vi "Control Panel.vi"(8 "error in (no error)":errorcluster, 11 "Fake MicrowaveAmp in":refnum<class "MicrowaveAmp.lvclass">) -> (0 "error out":errorcluster, 3 "Fake MicrowaveAmp out":refnum<class "MicrowaveAmp.lvclass">)   [LabVIEW 2009, in "MicrowaveAmp.lvclass"]
doc: "(Dynamic) A user-level application that simulates the physical front panel of the Instrument. Provide the user with buttons to manually control features of the instrument, and provide indicators of its current state."
uses:
  MicrowaveAmp.lvclass
  Utility Classes/Scannable/Scannable.lvclass
  MicrowaveAmp.lvclass/MicrowaveAmp.ctl
panel:
  in  "Copy actual to set":bool
  in  "Populate fields with member data":bool
  in  "Read Remaining Time Delay":bool
  in  "Read Amplifier Status/Mode":bool
  in  "Standby":bool
  in  "stop":bool
  out "Mode":u16(ring) items=["SLEEP", "WARM-UP", "STANDBY", "OPERATE", "FAULT"]
  in  "Operate":bool
  in  "Read Reverse Power Out (W)":bool
  in  "Read Reverse Power Out (dBm)":bool
  in  "Read Forward Power Out (W)":bool
  in  "Read Forward Power out (dBm)":bool
  in  "Read Gain":bool
  in  "Set Gain":bool
  out "Remaining Heater Delay Time":dbl[unit]
  out "Reverse Power Out (dBm)":dbl
  out "Reverse Power Out (W)":dbl[unit]
  out "Forward Power Out (dBm)":dbl
  out "Forward Power Out (W)":dbl[unit]
  out "Gain (%)":dbl
  in  "GainSet":dbl
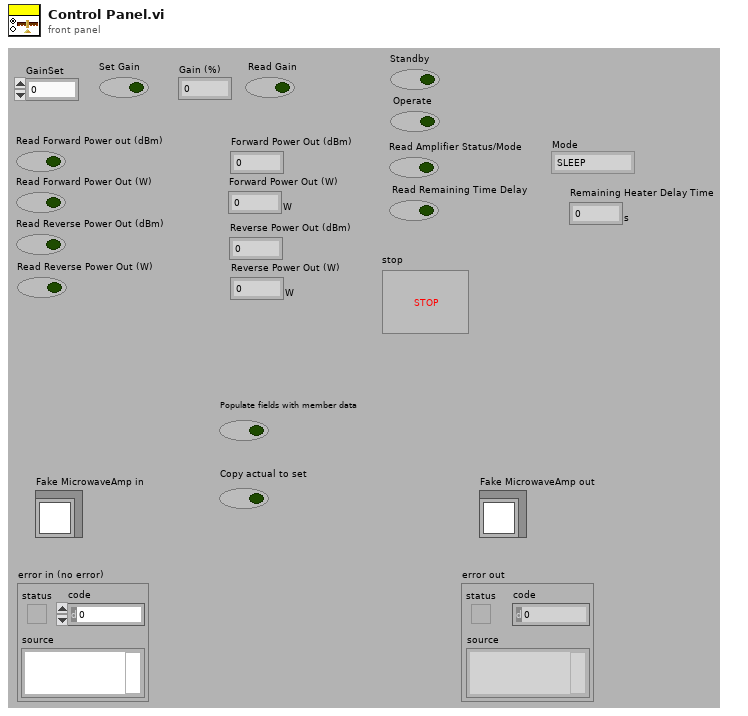
[diagram p1: front panel]
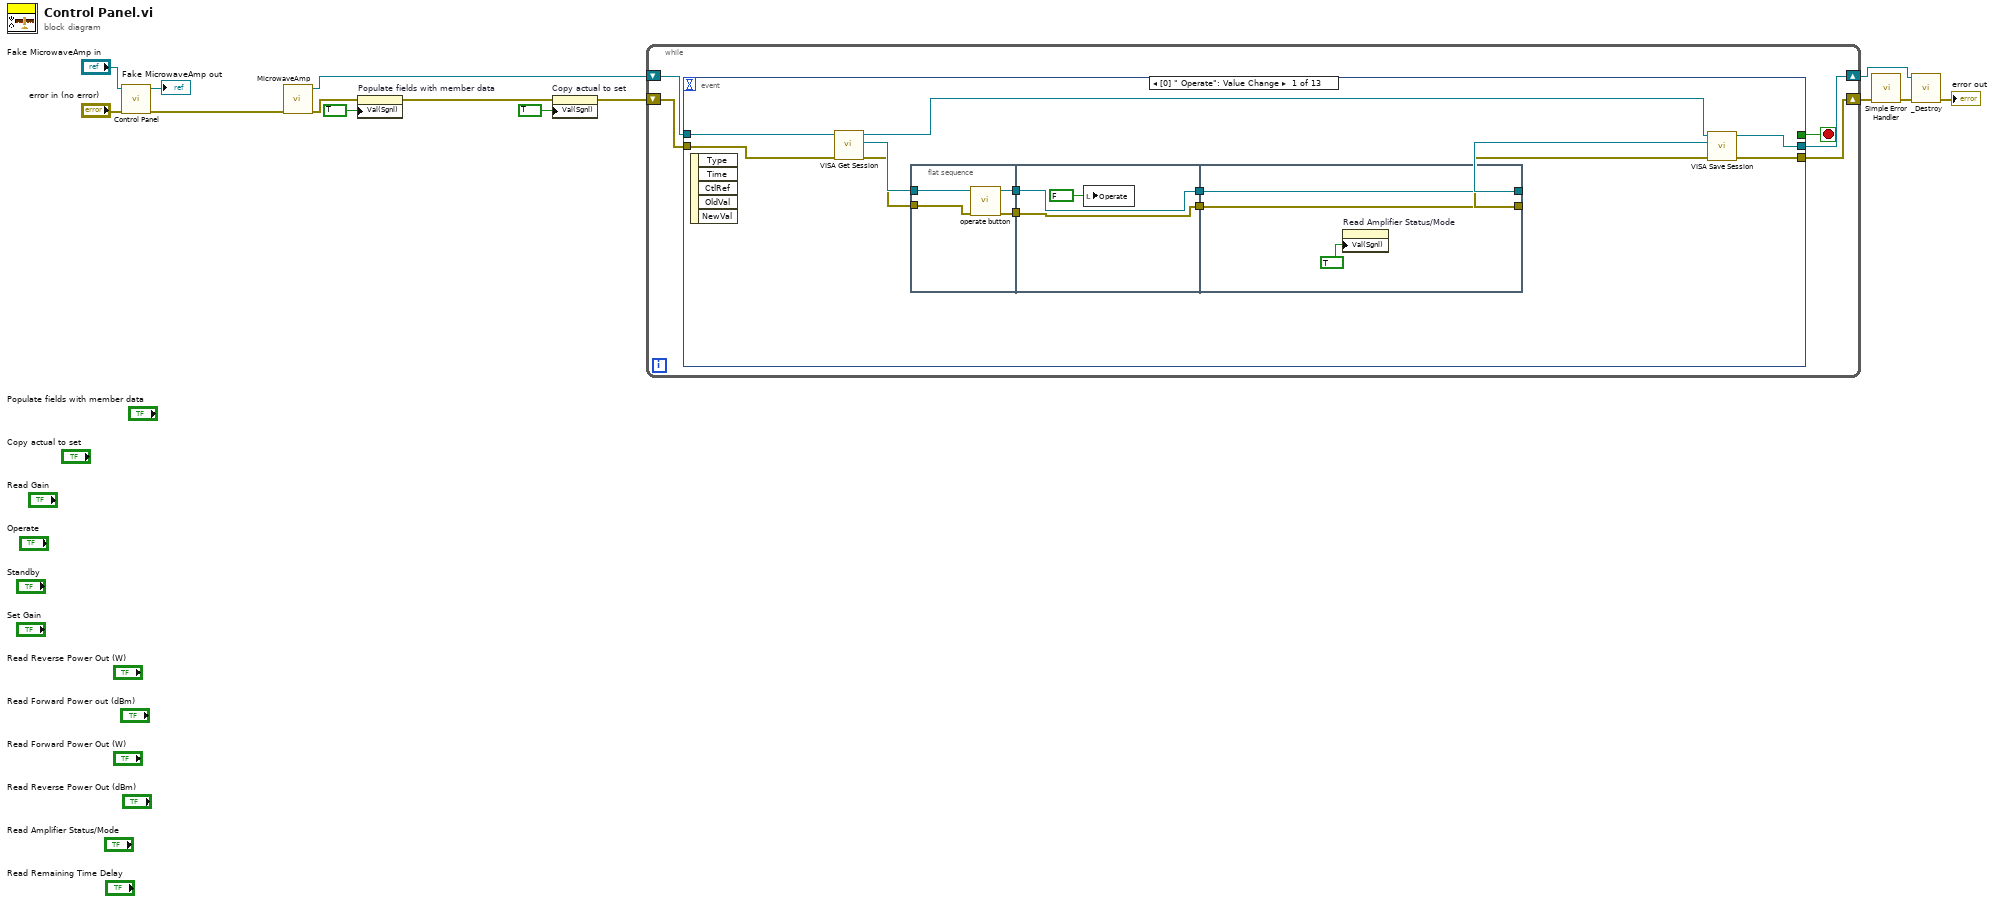
[diagram p0: block diagram]
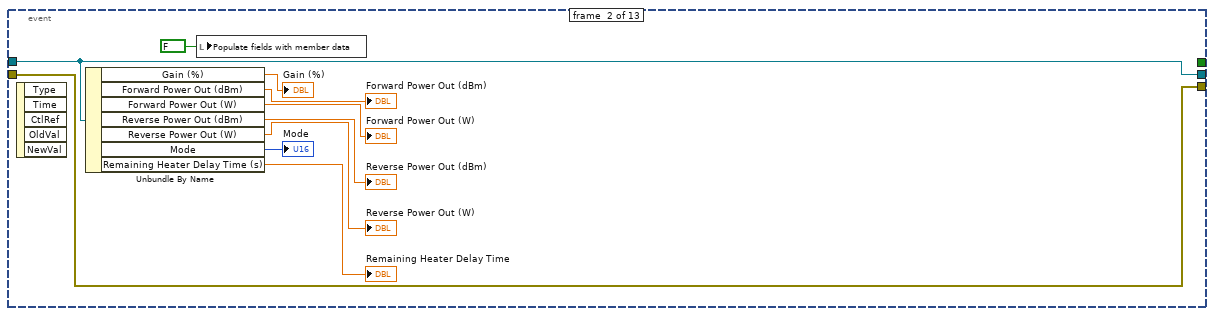
[diagram p2: hidden frame]
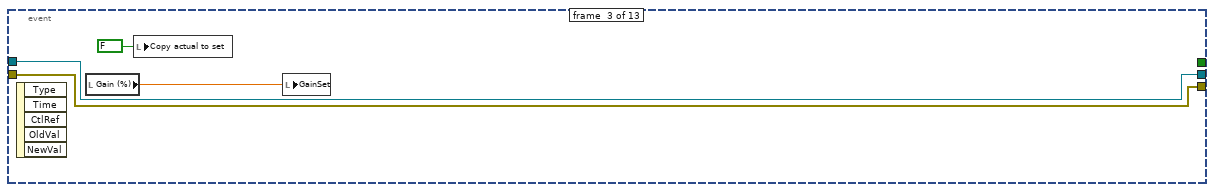
[diagram p3: hidden frame]
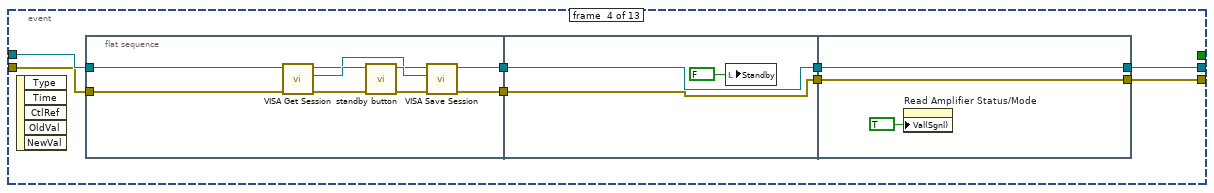
[diagram p4: hidden frame]
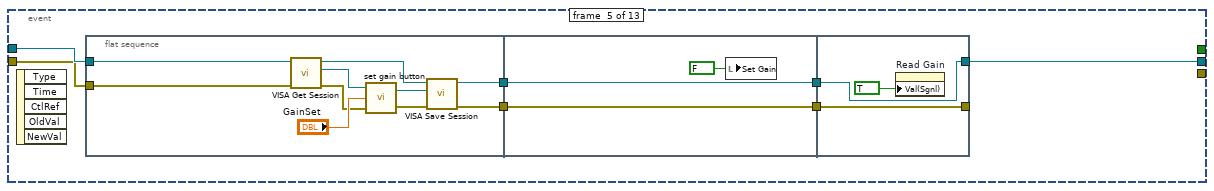
[diagram p5: hidden frame]
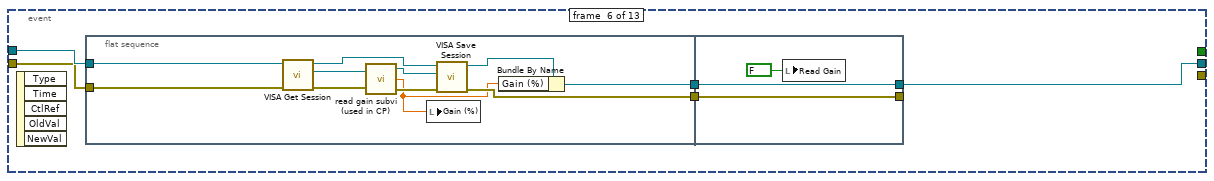
[diagram p6: hidden frame]
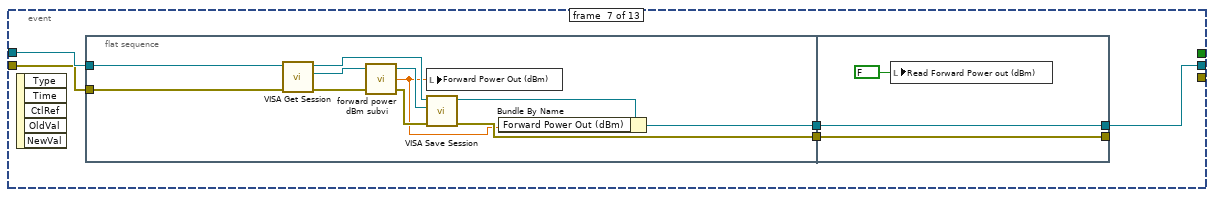
[diagram p7: hidden frame]
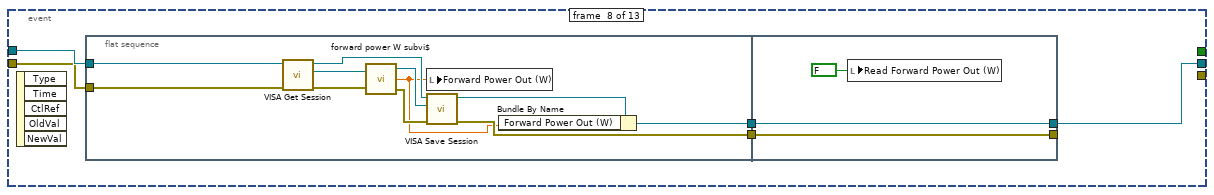
[diagram p8: hidden frame]
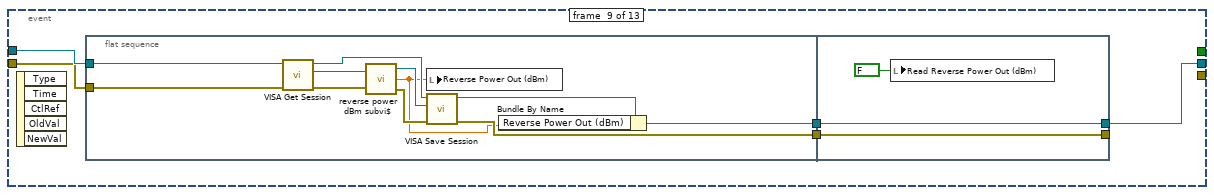
[diagram p9: hidden frame]
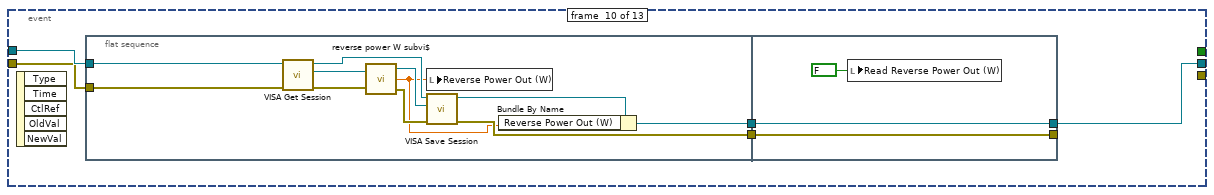
[diagram p10: hidden frame]
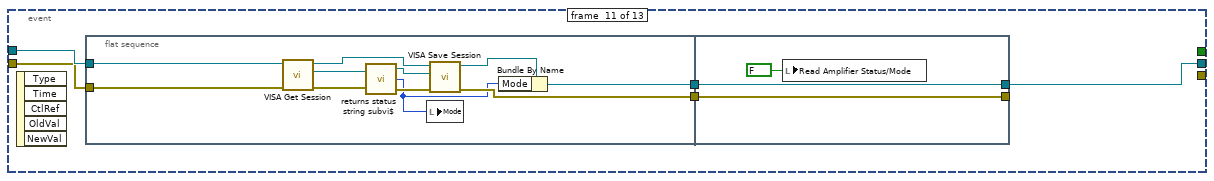
[diagram p11: hidden frame]
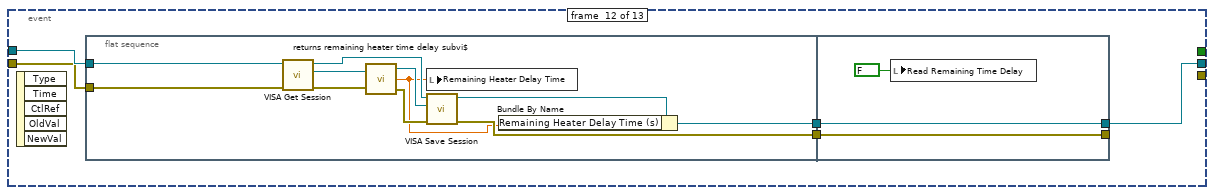
[diagram p12: hidden frame]
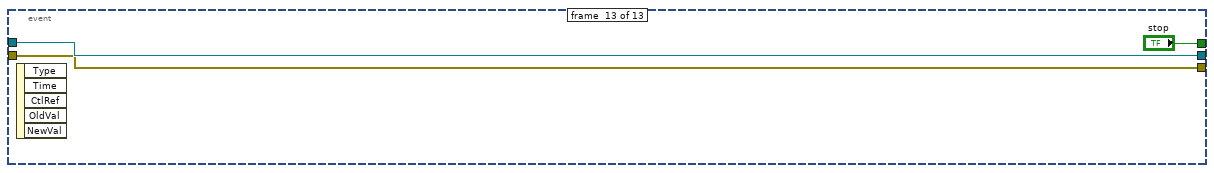
[diagram p13: hidden frame]
diagram:
  n1 = call-parent "Control Panel.vi"("error in (no error)"="error in (no error)", "Instrument in"="Fake MicrowaveAmp in") -> ("error out"=w9:errorcluster, "Instrument out"=→"Fake MicrowaveAmp out":refnum<class "MicrowaveAmp.lvclass">)  [unwired: 8 in]
  n2 = call "MicrowaveAmp.vi"("error in (no error)"=w9) -> ("error out"=w10:errorcluster, "MicrowaveAmp out"=w1:refnum<class "MicrowaveAmp.lvclass">)  [unwired: 9 in]
  n3 = property on="Populate fields with member data" class="Bool (strict)"(error in=w10, "Val(Sgnl)"=TRUE ("Value (Signaling)")) -> (error out=w11:errorcluster)  [unwired: 1 in, 1 out]
  n4 = property on="Copy actual to set" class="Bool (strict)"(error in=w11, "Val(Sgnl)"=TRUE ("Value (Signaling)")) -> (error out=w2:errorcluster)  [unwired: 1 in, 1 out]
  n5 = while {
    shift-right: [w19] -> w5
    shift-left: w2 -> [w16]
    shift-right: [w17] -> w8
    shift-left: w1 -> [w15]
    stop <- w18 stop-if-true
    n6 = event shown="[0] \" Operate\": Value Change" {
      selector: _ -> [_ _ _ _ _ _ _ _ _ _ _ _ _]
      dyn-events: _ -> [_ _ _ _ _ _ _ _ _ _ _ _ _]
      timeout: _ -> [_ _ _ _ _ _ _ _ _ _ _ _ _]
      tunnel: w16 -> [w23 w52 w55 w59 w83 w105 w122 w141 w160 w179 w198 w219 w236]
      tunnel: [w25 w52 w55 w63 _ _ _ _ _ _ _ _ w236] -> w19
      tunnel: [_ _ _ _ _ _ _ _ _ _ _ _ "stop"] -> w18
      tunnel: w15 -> [w29 w51 w56 w60 w84 w106 w125 w144 w163 w182 w201 w220 w237]
      tunnel: [w26 w51 w56 w61 w82 w104 w124 w143 w162 w181 w200 w218 w237] -> w17
      event #0 {
        n7 = event-data() -> ()  [unwired: 1 in, 5 out]
        n8 = call-dynamic "VISA Get Session.vi"("error in (no error)"=w23, "Instrument.lvclass in"=w29) -> ("error out"=w22:errorcluster, "VISA Resource Name"=w30:refnum<visa-resource-name>, "Instrument.lvclass out"=w27:refnum<class "MicrowaveAmp.lvclass">)  [unwired: 7 out]
        n9 = flat-sequence {
          tunnel: [w36] -> w32
          tunnel: [w35] -> w31
          tunnel: w22 -> [w34]
          tunnel: w30 -> [w33]
          tunnel: w32 -> [w38]
          tunnel: w31 -> [w37]
          tunnel: [w38] -> w21
          tunnel: [w37] -> w20
          tunnel: [w41] -> w24
          tunnel: [w42] -> w28
          tunnel: w21 -> [w42]
          tunnel: w20 -> [w41]
          frame #0 {
            n10 = call "operate button.vi"("error in (no error)"=w34, "VISA resource name"=w33) -> ("error out"=w35:errorcluster, "VISA resource name out"=w36:refnum<visa-resource-name>)  [unwired: 8 in]
          }
          frame #1 {
            n11 = local write "Operate"(FALSE ("Operate")) -> ()
          }
          frame #2 {
            n12 = property on="Read Amplifier Status/Mode" class="Bool (strict)"("Val(Sgnl)"=TRUE ("Value (Signaling)")) -> ()  [unwired: 2 in, 2 out]
          }
        }
        n13 = call-dynamic "VISA Save Session.vi"("error in (no error)"=w24, "VISA Resource Name"=w28, "Instrument.lvclass in"=w27) -> ("error out"=w25:errorcluster, "Instrument.lvclass out"=w26:refnum<class "MicrowaveAmp.lvclass">)  [unwired: 7 out]
      }
      event #1 {
        n14 = event-data() -> ()  [unwired: 1 in, 5 out]
        n15 = Unbundle By Name(w51) -> ("Gain (%)"=→"Gain (%)":dbl, "Forward Power Out (dBm)"=→"Forward Power Out (dBm)":dbl, "Forward Power Out (W)"=→"Forward Power Out (W)":dbl[unit], "Reverse Power Out (dBm)"=→"Reverse Power Out (dBm)":dbl, "Reverse Power Out (W)"=→"Reverse Power Out (W)":dbl[unit], "Mode"=→"Mode":u16, "Remaining Heater Delay Time (s)"=→"Remaining Heater Delay Time":dbl[unit])
        n16 = local write "Populate fields with member data"(FALSE ("Populate fields with member data")) -> ()
      }
      event #2 {
        n17 = event-data() -> ()  [unwired: 1 in, 5 out]
        n18 = local read "Gain (%)"() -> (w53:dbl)
        n19 = local write "Copy actual to set"(FALSE ("Copy actual to set")) -> ()
        n20 = local write "GainSet"(w53) -> ()
      }
      event #3 {
        n21 = event-data() -> ()  [unwired: 1 in, 5 out]
        n22 = flat-sequence {
          tunnel: [w72] -> w64
          tunnel: [w71] -> w62
          tunnel: w60 -> [w69]
          tunnel: w59 -> [w68]
          tunnel: w64 -> [w75]
          tunnel: w62 -> [w74]
          tunnel: [w75] -> w58
          tunnel: [w74] -> w57
          tunnel: [w78] -> w61
          tunnel: [w79] -> w63
          tunnel: w58 -> [w79]
          tunnel: w57 -> [w78]
          frame #0 {
            n23 = call-dynamic "VISA Get Session.vi"("error in (no error)"=w68, "Instrument.lvclass in"=w69) -> ("error out"=w67:errorcluster, "VISA Resource Name"=w66:refnum<visa-resource-name>, "Instrument.lvclass out"=w65:refnum<class "MicrowaveAmp.lvclass">)  [unwired: 7 out]
            n24 = call "standby button.vi"("error in (no error)"=w67, "VISA resource name"=w66) -> ("error out"=w70:errorcluster, "VISA resource name out"=w73:refnum<visa-resource-name>)  [unwired: 8 in]
            n25 = call-dynamic "VISA Save Session.vi"("error in (no error)"=w70, "VISA Resource Name"=w73, "Instrument.lvclass in"=w65) -> ("error out"=w72:errorcluster, "Instrument.lvclass out"=w71:refnum<class "MicrowaveAmp.lvclass">)  [unwired: 7 out]
          }
          frame #1 {
            n26 = local write "Standby"(FALSE ("Operate")) -> ()
          }
          frame #2 {
            n27 = property on="Read Amplifier Status/Mode" class="Bool (strict)"("Val(Sgnl)"=TRUE ("Value (Signaling)")) -> ()  [unwired: 2 in, 2 out]
          }
        }
      }
      event #4 {
        n28 = event-data() -> ()  [unwired: 1 in, 5 out]
        n29 = flat-sequence {
          tunnel: [w89] -> w86
          tunnel: w84 -> [w95]
          tunnel: w83 -> [w94]
          tunnel: [w92] -> w80
          tunnel: w86 -> [w98]
          tunnel: [w98] -> w85
          tunnel: [w97] -> w81
          tunnel: w80 -> [w97]
          tunnel: [w102] -> _
          tunnel: w85 -> [w102]
          tunnel: [w100] -> w82
          tunnel: w81 -> [w100]
          frame #0 {
            n30 = call-dynamic "VISA Get Session.vi"("error in (no error)"=w94, "Instrument.lvclass in"=w95) -> ("error out"=w91:errorcluster, "VISA Resource Name"=w87:refnum<visa-resource-name>, "Instrument.lvclass out"=w93:refnum<class "MicrowaveAmp.lvclass">)  [unwired: 7 out]
            n31 = call "set gain button.vi"("error in (no error)"=w91, "Gain"="GainSet", "VISA resource name"=w87) -> ("error out"=w90:errorcluster, "VISA resource name out"=w88:refnum<visa-resource-name>)
            n32 = call-dynamic "VISA Save Session.vi"("error in (no error)"=w90, "VISA Resource Name"=w88, "Instrument.lvclass in"=w93) -> ("error out"=w89:errorcluster, "Instrument.lvclass out"=w92:refnum<class "MicrowaveAmp.lvclass">)  [unwired: 7 out]
          }
          frame #1 {
            n33 = local write "Set Gain"(FALSE ("Set Gain")) -> ()
          }
          frame #2 {
            n34 = property on="Read Gain" class="Bool (strict)"("Val(Sgnl)"=TRUE ("Value (Signaling)")) -> ()  [unwired: 2 in, 2 out]
          }
        }
      }
      event #5 {
        n35 = event-data() -> ()  [unwired: 1 in, 5 out]
        n36 = flat-sequence {
          tunnel: [w114] -> w107
          tunnel: w106 -> [w118]
          tunnel: w105 -> [w117]
          tunnel: [w108] -> w103
          tunnel: [w120] -> _
          tunnel: w107 -> [w120]
          tunnel: [w119] -> w104
          tunnel: w103 -> [w119]
          frame #0 {
            n37 = call-dynamic "VISA Get Session.vi"("error in (no error)"=w117, "Instrument.lvclass in"=w118) -> ("error out"=w116:errorcluster, "VISA Resource Name"=w113:refnum<visa-resource-name>, "Instrument.lvclass out"=w111:refnum<class "MicrowaveAmp.lvclass">)  [unwired: 7 out]
            n38 = call "read gain subvi (used in CP).vi"("VISA resource name"=w113, "error in (no error)"=w116) -> ("VISA resource name out"=w112:refnum<visa-resource-name>, "Gain (%)"=w110:dbl, "error out"=w115:errorcluster)
            n39 = local write "Gain (%)"(w110) -> ()
            n40 = call-dynamic "VISA Save Session.vi"("error in (no error)"=w115, "VISA Resource Name"=w112, "Instrument.lvclass in"=w111) -> ("error out"=w114:errorcluster, "Instrument.lvclass out"=w109:refnum<class "MicrowaveAmp.lvclass">)  [unwired: 7 out]
            n41 = Bundle By Name(cluster=w109, "Gain (%)"=w110) -> (w108:refnum<class "MicrowaveAmp.lvclass">)
          }
          frame #1 {
            n42 = local write "Read Gain"(FALSE ("Read Gain")) -> ()
          }
        }
      }
      event #6 {
        n43 = event-data() -> ()  [unwired: 1 in, 5 out]
        n44 = flat-sequence {
          tunnel: [w132] -> w126
          tunnel: w125 -> [w137]
          tunnel: [w127] -> w123
          tunnel: w122 -> [w135]
          tunnel: [w140] -> _
          tunnel: w126 -> [w140]
          tunnel: [w138] -> w124
          tunnel: w123 -> [w138]
          frame #0 {
            n45 = call-dynamic "VISA Get Session.vi"("error in (no error)"=w135, "Instrument.lvclass in"=w137) -> ("error out"=w134:errorcluster, "VISA Resource Name"=w131:refnum<visa-resource-name>, "Instrument.lvclass out"=w136:refnum<class "MicrowaveAmp.lvclass">)  [unwired: 7 out]
            n46 = call "forward power dBm subvi.vi"("error in (no error)"=w134, "VISA resource name"=w131) -> ("error out"=w133:errorcluster, "forward power (dBm)"=w129:dbl, "VISA resource name out"=w130:refnum<visa-resource-name>)  [unwired: 1 in]
            n47 = local write "Forward Power Out (dBm)"(w129) -> ()
            n48 = call-dynamic "VISA Save Session.vi"("error in (no error)"=w133, "VISA Resource Name"=w130, "Instrument.lvclass in"=w136) -> ("error out"=w132:errorcluster, "Instrument.lvclass out"=w128:refnum<class "MicrowaveAmp.lvclass">)  [unwired: 7 out]
            n49 = Bundle By Name(cluster=w128, "Forward Power Out (dBm)"=w129) -> (w127:refnum<class "MicrowaveAmp.lvclass">)
          }
          frame #1 {
            n50 = local write "Read Forward Power out (dBm)"(FALSE ("Read Forward Power out (dBm)")) -> ()
          }
        }
      }
      event #7 {
        n51 = event-data() -> ()  [unwired: 1 in, 5 out]
        n52 = flat-sequence {
          tunnel: [w150] -> w145
          tunnel: w144 -> [w155]
          tunnel: [w146] -> w142
          tunnel: w141 -> [w153]
          tunnel: [w159] -> _
          tunnel: w145 -> [w159]
          tunnel: [w157] -> w143
          tunnel: w142 -> [w157]
          frame #0 {
            n53 = call-dynamic "VISA Get Session.vi"("error in (no error)"=w153, "Instrument.lvclass in"=w155) -> ("error out"=w152:errorcluster, "VISA Resource Name"=w156:refnum<visa-resource-name>, "Instrument.lvclass out"=w154:refnum<class "MicrowaveAmp.lvclass">)  [unwired: 7 out]
            n54 = call "forward power W subvi$.vi"("VISA resource name"=w156, "error in (no error)"=w152) -> ("VISA resource name out"=w149:refnum<visa-resource-name>, "foward power (W)"=w148:dbl[unit], "error out"=w151:errorcluster)
            n55 = local write "Forward Power Out (W)"(w148) -> ()
            n56 = call-dynamic "VISA Save Session.vi"("error in (no error)"=w151, "VISA Resource Name"=w149, "Instrument.lvclass in"=w154) -> ("error out"=w150:errorcluster, "Instrument.lvclass out"=w147:refnum<class "MicrowaveAmp.lvclass">)  [unwired: 7 out]
            n57 = Bundle By Name(cluster=w147, "Forward Power Out (W)"=w148) -> (w146:refnum<class "MicrowaveAmp.lvclass">)
          }
          frame #1 {
            n58 = local write "Read Forward Power Out (W)"(FALSE ("Read Forward Power Out (W)")) -> ()
          }
        }
      }
      event #8 {
        n59 = event-data() -> ()  [unwired: 1 in, 5 out]
        n60 = flat-sequence {
          tunnel: [w168] -> w164
          tunnel: w163 -> [w175]
          tunnel: [w165] -> w161
          tunnel: w160 -> [w173]
          tunnel: [w177] -> _
          tunnel: w164 -> [w177]
          tunnel: [w176] -> w162
          tunnel: w161 -> [w176]
          frame #0 {
            n61 = call-dynamic "VISA Get Session.vi"("error in (no error)"=w173, "Instrument.lvclass in"=w175) -> ("error out"=w170:errorcluster, "VISA Resource Name"=w172:refnum<visa-resource-name>, "Instrument.lvclass out"=w174:refnum<class "MicrowaveAmp.lvclass">)  [unwired: 7 out]
            n62 = call "reverse power dBm subvi$.vi"("VISA resource name 2"=w172, "error in (no error)"=w170) -> ("VISA resource name out 2"=w171:refnum<visa-resource-name>, "reverse power (dBm)"=w167:dbl, "error out"=w169:errorcluster)
            n63 = local write "Reverse Power Out (dBm)"(w167) -> ()
            n64 = call-dynamic "VISA Save Session.vi"("error in (no error)"=w169, "VISA Resource Name"=w171, "Instrument.lvclass in"=w174) -> ("error out"=w168:errorcluster, "Instrument.lvclass out"=w166:refnum<class "MicrowaveAmp.lvclass">)  [unwired: 7 out]
            n65 = Bundle By Name(cluster=w166, "Reverse Power Out (dBm)"=w167) -> (w165:refnum<class "MicrowaveAmp.lvclass">)
          }
          frame #1 {
            n66 = local write "Read Reverse Power Out (dBm)"(FALSE ("Read Reverse Power Out (dBm)")) -> ()
          }
        }
      }
      event #9 {
        n67 = event-data() -> ()  [unwired: 1 in, 5 out]
        n68 = flat-sequence {
          tunnel: [w189] -> w183
          tunnel: w182 -> [w194]
          tunnel: [w185] -> w180
          tunnel: w179 -> [w192]
          tunnel: [w196] -> _
          tunnel: w183 -> [w196]
          tunnel: [w195] -> w181
          tunnel: w180 -> [w195]
          frame #0 {
            n69 = call-dynamic "VISA Get Session.vi"("error in (no error)"=w192, "Instrument.lvclass in"=w194) -> ("error out"=w191:errorcluster, "VISA Resource Name"=w188:refnum<visa-resource-name>, "Instrument.lvclass out"=w193:refnum<class "MicrowaveAmp.lvclass">)  [unwired: 7 out]
            n70 = call "reverse power W subvi$.vi"("VISA resource name"=w188, "error in (no error)"=w191) -> ("VISA resource name out"=w187:refnum<visa-resource-name>, "Reverse Power (W)"=w184:dbl[unit], "error out"=w190:errorcluster)
            n71 = local write "Reverse Power Out (W)"(w184) -> ()
            n72 = call-dynamic "VISA Save Session.vi"("error in (no error)"=w190, "VISA Resource Name"=w187, "Instrument.lvclass in"=w193) -> ("error out"=w189:errorcluster, "Instrument.lvclass out"=w186:refnum<class "MicrowaveAmp.lvclass">)  [unwired: 7 out]
            n73 = Bundle By Name(cluster=w186, "Reverse Power Out (W)"=w184) -> (w185:refnum<class "MicrowaveAmp.lvclass">)
          }
          frame #1 {
            n74 = local write "Read Reverse Power Out (W)"(FALSE ("Read Reverse Power Out (W)")) -> ()
          }
        }
      }
      event #10 {
        n75 = event-data() -> ()  [unwired: 1 in, 5 out]
        n76 = flat-sequence {
          tunnel: [w208] -> w202
          tunnel: w201 -> [w213]
          tunnel: [w204] -> w199
          tunnel: w198 -> [w211]
          tunnel: [w216] -> _
          tunnel: w202 -> [w216]
          tunnel: [w214] -> w200
          tunnel: w199 -> [w214]
          frame #0 {
            n77 = call-dynamic "VISA Get Session.vi"("error in (no error)"=w211, "Instrument.lvclass in"=w213) -> ("error out"=w210:errorcluster, "VISA Resource Name"=w207:refnum<visa-resource-name>, "Instrument.lvclass out"=w212:refnum<class "MicrowaveAmp.lvclass">)  [unwired: 7 out]
            n78 = call "returns status string subvi$.vi"("VISA resource name"=w207, "error in (no error)"=w210) -> ("VISA resource name out"=w206:refnum<visa-resource-name>, "Mode"=w203:u16, "error out"=w209:errorcluster)
            n79 = local write "Mode"(w203) -> ()
            n80 = call-dynamic "VISA Save Session.vi"("error in (no error)"=w209, "VISA Resource Name"=w206, "Instrument.lvclass in"=w212) -> ("error out"=w208:errorcluster, "Instrument.lvclass out"=w205:refnum<class "MicrowaveAmp.lvclass">)  [unwired: 7 out]
            n81 = Bundle By Name(cluster=w205, "Mode"=w203) -> (w204:refnum<class "MicrowaveAmp.lvclass">)
          }
          frame #1 {
            n82 = local write "Read Amplifier Status/Mode"(FALSE ("Read Amplifier Status")) -> ()
          }
        }
      }
      event #11 {
        n83 = event-data() -> ()  [unwired: 1 in, 5 out]
        n84 = flat-sequence {
          tunnel: [w227] -> w221
          tunnel: w220 -> [w232]
          tunnel: w219 -> [w231]
          tunnel: [w222] -> w217
          tunnel: [w235] -> _
          tunnel: w221 -> [w235]
          tunnel: [w233] -> w218
          tunnel: w217 -> [w233]
          frame #0 {
            n85 = call-dynamic "VISA Get Session.vi"("error in (no error)"=w231, "Instrument.lvclass in"=w232) -> ("error out"=w229:errorcluster, "VISA Resource Name"=w226:refnum<visa-resource-name>, "Instrument.lvclass out"=w230:refnum<class "MicrowaveAmp.lvclass">)  [unwired: 7 out]
            n86 = call "returns remaining heater time delay subvi$.vi"("VISA resource name"=w226, "error in (no error)"=w229) -> ("VISA resource name out"=w225:refnum<visa-resource-name>, "Heater delay time (s)"=w224:dbl[unit], "error out"=w228:errorcluster)
            n87 = local write "Remaining Heater Delay Time"(w224) -> ()
            n88 = call-dynamic "VISA Save Session.vi"("error in (no error)"=w228, "VISA Resource Name"=w225, "Instrument.lvclass in"=w230) -> ("error out"=w227:errorcluster, "Instrument.lvclass out"=w223:refnum<class "MicrowaveAmp.lvclass">)  [unwired: 7 out]
            n89 = Bundle By Name(cluster=w223, "Remaining Heater Delay Time (s)"=w224) -> (w222:refnum<class "MicrowaveAmp.lvclass">)
          }
          frame #1 {
            n90 = local write "Read Remaining Time Delay"(FALSE ("Read Remaining Time Delay")) -> ()
          }
        }
      }
      event #12 {
        n91 = event-data() -> ()  [unwired: 1 in, 5 out]
      }
    }
  }
  n92 = call <vilib>:"Simple Error Handler.vi"("error in (no error)"=w5) -> ("error out"=w7:errorcluster)  [unwired: 1 in, 7 out]
  n93 = call-dynamic "_Destroy.vi"("error in (no error)"=w7, "Instrument in"=w8) -> ("error out"=→"error out":errorcluster)  [unwired: 9 out]
